vi "Process Set Point Command (SubVI).vi"(4 "Setpoint":dbl format="%_4g", 6 "Address":string, 8 "error in (no error)":errorcluster, 11 "VISA Refnum in":refnum<visa-resource-name>) -> (0 "error out":errorcluster, 2 "Setpoint Value Out":string, 3 "VISA Refnum out":refnum<visa-resource-name>)   [LabVIEW 2020]
doc: "Reads/writes setpoint value from/to the instrument. To read current setpoint value wire to the \"Setpoint\" terminal -1."
uses:
  <vilib>/Instr/_visa.llb/VISA Flush IO Buffer Mask.ctl
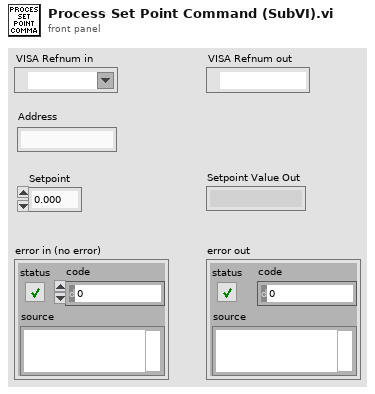
[diagram p1: front panel]
types:
  T1 = typedef "VISA Flush IO Buffer Mask.ctl" = u16
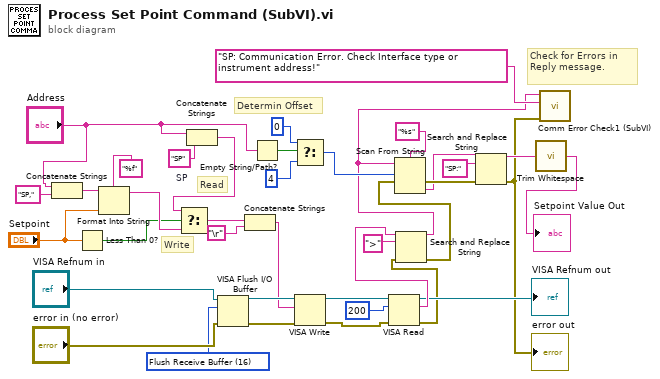
[diagram p0: block diagram]
diagram:
  w26 = "SP"  # SP
  w27 = T1 16 items=["Flush Receive Buffer"=16, "Write Transmit Buffer to Device"=32, "Flush Receive Buffer (No I/O)"=64, "Flush Transmit Buffer"=128] ("Mask")
  # "Write"
  # "Read"
  # "Check for Errors in Reply message."
  # "Determin Offset"
  n1 = Concatenate Strings("Address", "SP,") -> (w5:string)
  n2 = Less Than 0?(x="Setpoint") -> (x < 0?=w1:bool)
  n3 = Format Into String(format string="%f", initial string=w5, "Setpoint") -> (resulting string=w3:string)  [unwired: 1 in, 1 out]
  n4 = Concatenate Strings("Address", w26) -> (w10:string)
  n5 = Select(t=w10, s=w1, f=w3) -> (s? t:f=w9:string)
  n6 = VISA Flush I/O Buffer(VISA resource name="VISA Refnum in", mask (16)=w27, error in (no error)="error in (no error)") -> (VISA resource name out=w32:refnum<visa-resource-name>, error out=w8:errorcluster)
  n7 = Concatenate Strings(w9, "\r") -> (w31:string)
  n8 = Empty String/Path?(string/path="Address") -> (empty?=w22:bool)
  n9 = Select(t=u32 0, s=w22, f=u32 4) -> (s? t:f=w15:u32)
  n10 = VISA Write(VISA resource name=w32, write buffer=w31, error in (no error)=w8) -> (VISA resource name out=w34:refnum<visa-resource-name>, error out=w38:errorcluster)  [unwired: 1 out]
  n11 = VISA Read(VISA resource name=w34, byte count=u32 200, error in (no error)=w38) -> (VISA resource name out=→"VISA Refnum out":refnum<visa-resource-name>, read buffer=w37:string, error out=w18:errorcluster)  [unwired: 1 out]
  n12 = Search and Replace String(input string=w37, search string=">", error in=w18) -> (result string=w12:string, error out=w17:errorcluster)  [unwired: 5 in, 2 out]
  n13 = Scan From String(format string="%s", input string=w12, initial scan location=w15, error in=w17) -> (error out=w16:errorcluster, output 1=w14:string)  [unwired: 1 in, 2 out]
  n14 = Search and Replace String(input string=w14, search string="SP:", error in=w16) -> (result string=w24:string, error out=w11:errorcluster)  [unwired: 5 in, 2 out]
  "error out" <- w11
  n15 = call <vilib>:"Trim Whitespace.vi"("string"=w24) -> ("trimmed string"=→"Setpoint Value Out":string)  [unwired: 1 in]
  n16 = call "Comm Error Check1 (SubVI).vi"("error in (no error)"=w11, "Error Source String"="SP: Communication Error. Check Interface type or instrument address!", "result string"=w12) -> ()  [unwired: 9 in]
